vi "Jump Button Facade.vi"(0 "Data In":T4, 2 "Display State In":T2, 3 "Container State":T3) -> (6 "Data Out":T4, 7 "Display State Out":T2, 8 "Action":T1)   [LabVIEW 2009, in "Jump Button (System).xctl"]
uses:
  <vilib>/Navigation Controls/Jump Button System/Jump Button (System).xctl
  <vilib>/Navigation Controls/Jump Button System/Jump Button Data.ctl
  <vilib>/_xctls/Container State.ctl
  <vilib>/Navigation Controls/Jump Button System/Jump Button State.ctl
  <vilib>/_xctls/Action.ctl
  <vilib>/_xctls/XControlSupport.lvlib
  <vilib>/Navigation Controls/NI_Navigation.lvlib
panel:
  in  "Jump Button":bool
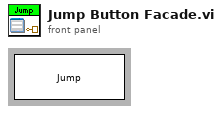
[diagram p1: front panel]
types:
  T1 = typedef "XControlSupport.lvlib/Action.ctl" = cluster{"Data Changed?":bool, "State Changed?":bool, "Action Name":string}
  T2 = typedef "Jump Button (System).xctl/Jump Button State.ctl" = cluster{"Button Text":string, "Absolute Path":path, "Relative Path":path}
  T3 = typedef "XControlSupport.lvlib/Container State.ctl" = cluster{"Indicator?":bool, "Run Mode?":bool, " Refnum":refnum<vi>}
  T4 = typedef "Jump Button (System).xctl/Jump Button Data.ctl" = bool
  T5 = cluster{"Button Text":string, "Absolute Path":path, "Relative Path":path}
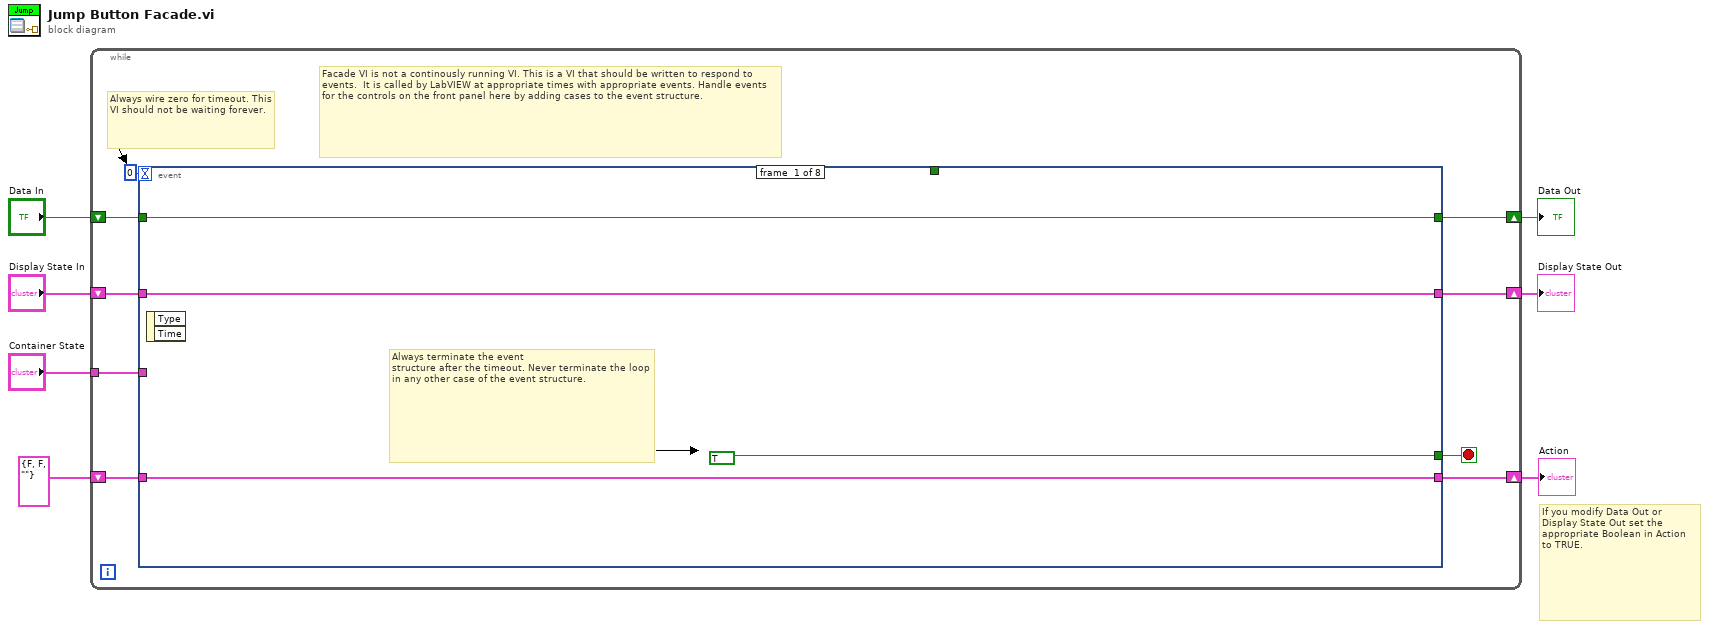
[diagram p0: block diagram]
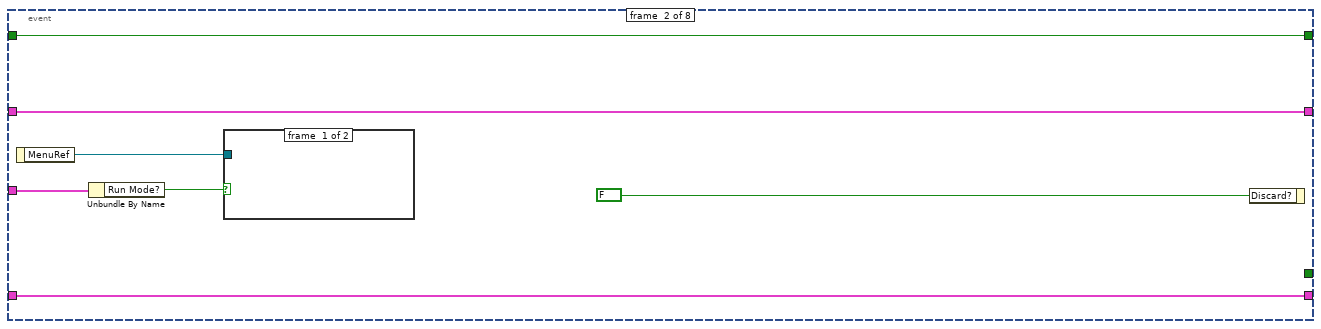
[diagram p2: hidden frame]
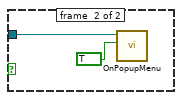
[diagram p3: hidden frame]
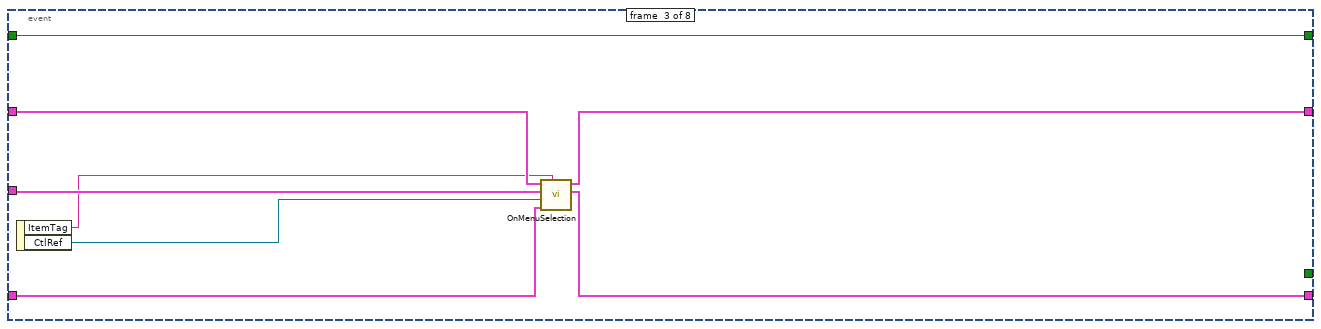
[diagram p4: hidden frame]
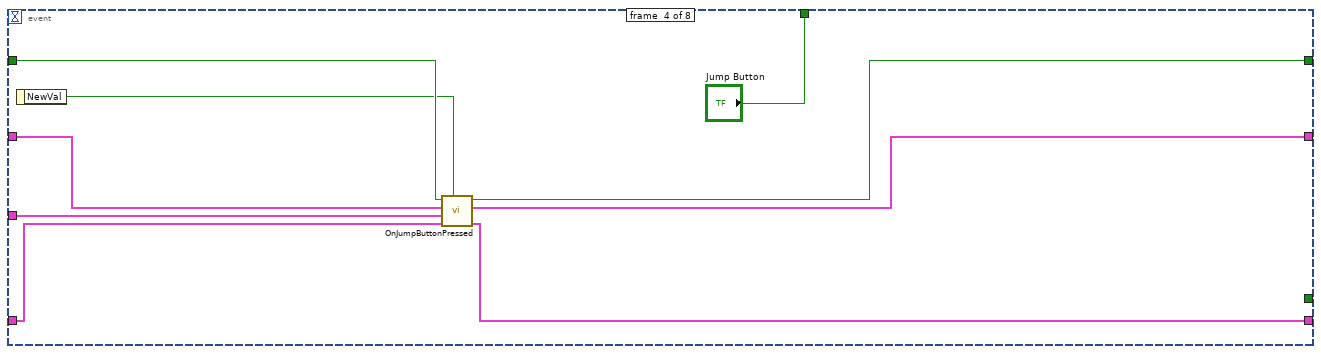
[diagram p5: hidden frame]
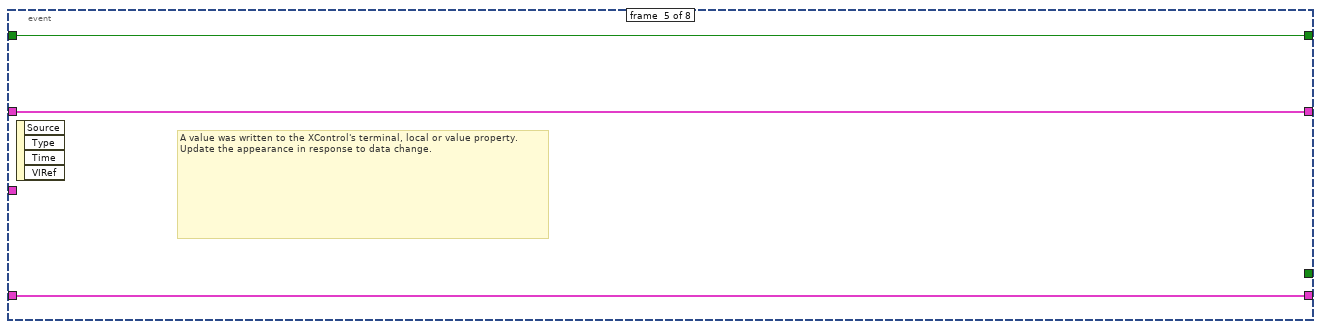
[diagram p6: hidden frame]
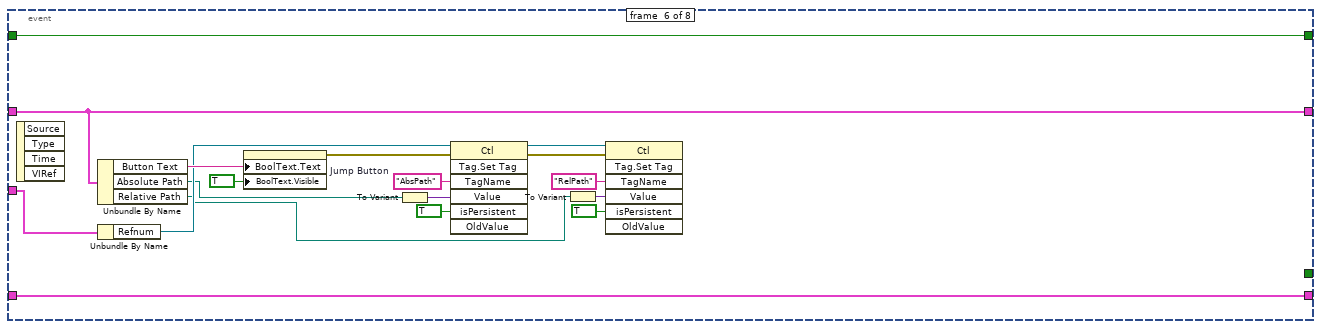
[diagram p7: hidden frame]
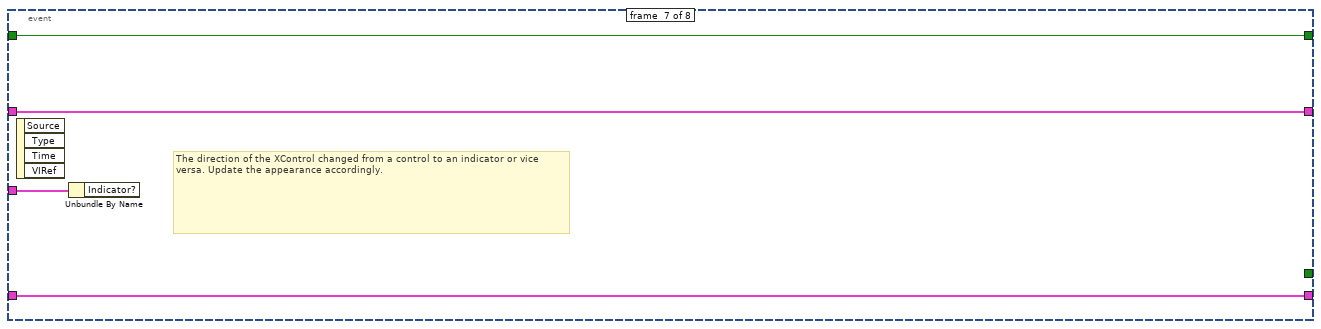
[diagram p8: hidden frame]
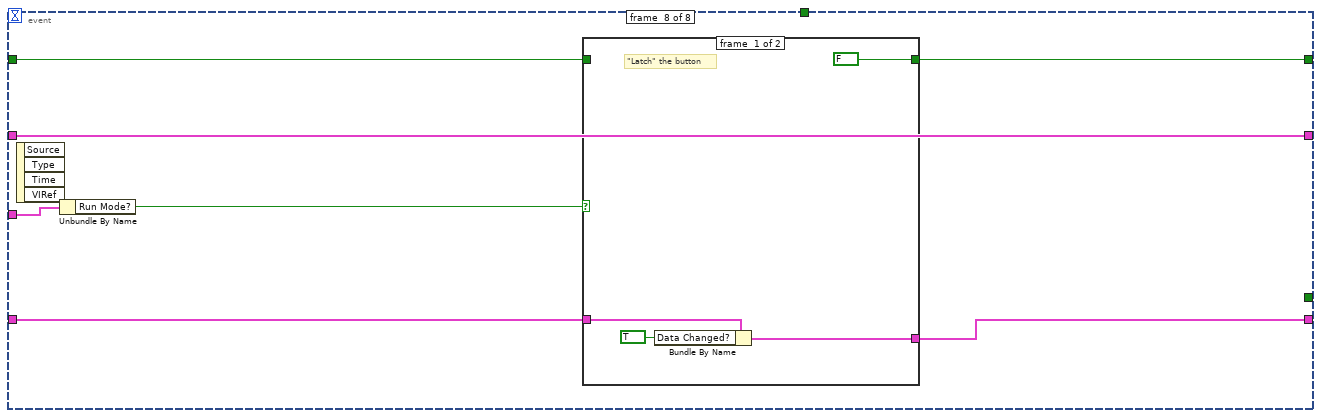
[diagram p9: hidden frame]
diagram:
  # "If you modify Data Out or\nDisplay State Out set the\nappropriate Boolean in Action\nto TRUE."
  n1 = while {
    shift-right: [w15] -> w4
    shift-left: "Display State In" -> [w16]
    tunnel: "Container State" -> [w12]
    shift-right: [w10] -> w7
    shift-left: "Data In" -> [w11]
    shift-right: [w8] -> w2
    shift-left: T1 {"Data Changed?"=FALSE, "State Changed?"=FALSE, "Action Name"=""} ("Action") -> [w9]
    stop <- w14 stop-if-true
    # "Facade VI is not a continously running VI. This is a VI that should be written to respond to events.  It is called by LabVIEW at appropriate times with appropriate events. Handle events for the controls on the front panel here by adding cases to the event structure."
    # "Always wire zero for timeout. This\nVI should not be waiting forever."
    n2 = event shown="[5] Display State Change" {
      selector: _ -> [_ _ _ _ _ _ _ _]
      dyn-events: _ -> [_ _ _ _ _ _ _ _]
      timeout: 0 -> [_ _ _ _ _ _ _ _]
      tunnel: w16 -> [w18 w26 w36 w42 w48 w65 w70 w77]
      tunnel: [w18 w26 w32 w39 w48 w65 w70 w77] -> w15
      tunnel: [TRUE _ _ _ _ _ _ _] -> w14
      tunnel: w12 -> [_ w24 w35 w44 _ w53 w71 w78]
      tunnel: w11 -> [w17 w27 w37 w43 w49 w67 w69 w72]
      tunnel: [w17 w27 w37 w41 w49 w67 w69 w75] -> w10
      tunnel: [w19 w25 w31 w38 w47 w64 w68 w73] -> w8
      tunnel: w9 -> [w19 w25 w33 w45 w47 w64 w68 w74]
      tunnel: [_ _ _ "Jump Button" _ _ _ _] -> _
      event #0 {
        # "Always terminate the event\nstructure after the timeout. Never terminate the loop in any other case of the event structure."
        n3 = event-data() -> ()  [unwired: 1 in, 2 out]
      }
      event #1 {
        n4 = event-data() -> ("MenuRef"=w22:refnum<k9>)  [unwired: 1 in]
        n5 = Unbundle By Name(w24) -> ("Run Mode?"=w21:bool)
        n6 = case shown="False" w21 {
          tunnel: w22 -> [_ w29]
          frame #0 {
          }
          frame #1 {
            n7 = call <vilib>:"OnPopupMenu.vi"("Configurable?"=TRUE, "MenuRef"=w29) -> ()  [unwired: 10 in]
          }
        }
        n8 = event-data("Discard?"=FALSE) -> ()  [unwired: 1 in, 1 out]
      }
      event #2 {
        n9 = event-data() -> ("ItemTag"=w30:string, "CtlRef"=w34:refnum<vi>)  [unwired: 1 in]
        n10 = call <vilib>:"OnMenuSelection.vi"("Tag"=w30, "Action In"=w33, "Button Reference"=w34, "Container State"=w35, "Display State In"=w36) -> ("Action Out"=w31:T1, "Display State Out"=w32:T5)  [unwired: 5 in]
      }
      event #3 {
        n11 = event-data() -> ("NewVal"=w40:bool)  [unwired: 1 in]
        n12 = call <vilib>:"OnJumpButtonPressed.vi"("NewVal"=w40, "action in"=w45, "container state in"=w44, "display state in"=w42, "data in"=w43) -> ("action out"=w38:T1, "display state out"=w39:T5, "data out"=w41:bool)  [unwired: 4 in]
      }
      event #4 {
        # "A value was written to the XControl's terminal, local or value property.\nUpdate the appearance in response to data change."
        n13 = event-data() -> ()  [unwired: 1 in, 4 out]
      }
      event #5 {
        n14 = event-data() -> ()  [unwired: 1 in, 4 out]
        n15 = Unbundle By Name(w65) -> ("Button Text"=w66:string, "Absolute Path"=w51:path, "Relative Path"=w50:path)
        n16 = Unbundle By Name(w53) -> ("Refnum"=w52:refnum<vi>)
        n17 = property on="Jump Button" class="Bool"("BoolText.Text"=w66, "BoolText.Visible"=TRUE ("Boolean Text.Visible")) -> (error out=w55:errorcluster)  [unwired: 2 in, 1 out]
        n18 = To Variant(anything=w51) -> (Variant=w62:variant)
        n19 = invoke class="Ctl" method="Tag.Set Tag"(reference=w52, error in=w55, "TagName"="AbsPath" ("Tag Name"), "Value"=w62, "isPersistent"=TRUE ("Is Persistent?")) -> (reference out=w60:refnum<vi>, error out=w59:errorcluster)  [unwired: 2 in, 5 out]
        n20 = To Variant(anything=w50) -> (Variant=w57:variant)
        n21 = invoke class="Ctl" method="Tag.Set Tag"(reference=w60, error in=w59, "TagName"="RelPath" ("Tag Name"), "Value"=w57, "isPersistent"=TRUE ("Is Persistent?")) -> ()  [unwired: 2 in, 7 out]
      }
      event #6 {
        # "The direction of the XControl changed from a control to an indicator or vice versa. Update the appearance accordingly."
        n22 = event-data() -> ()  [unwired: 1 in, 4 out]
        n23 = Unbundle By Name(w71) -> ()  [unwired: 1 out]
      }
      event #7 {
        n24 = event-data() -> ()  [unwired: 1 in, 4 out]
        n25 = Unbundle By Name(w78) -> ("Run Mode?"=w76:bool)
        n26 = case shown="False" w76 {
          tunnel: [T4 FALSE ("Data In") w83] -> w75
          tunnel: w74 -> [w81 w84]
          tunnel: [w79 w84] -> w73
          tunnel: w72 -> [_ w83]
          frame #0 {
            # "\"Latch\" the button"
            n27 = Bundle By Name(cluster=w81, "Data Changed?"=TRUE) -> (w79:T1)
          }
          frame #1 {
          }
        }
      }
    }
  }
  "Display State Out" <- w4
  "Data Out" <- w7
  "Action" <- w2
